vi "Parse XML.vi"(8 "error in (no error)":errorcluster, 10 "xml string":string) -> (0 "error out":errorcluster, 3 "xml out":T1)   [LabVIEW 2011]
uses:
  XML Structure - Cluster.ctl
  XML Tag Type - Enum.ctl
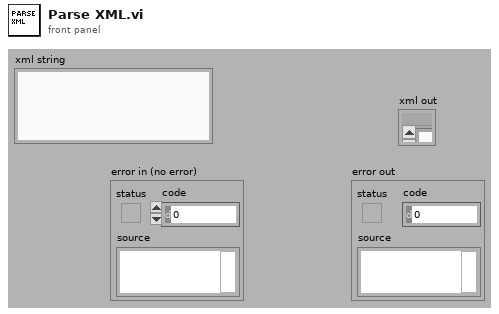
[diagram p1: front panel]
types:
  T1 = typedef "XML Structure - Cluster.ctl" = cluster{"tags":string[], "tag names":string[], "tag type":T2[], "offset":i32[], "close tag index":i32[], "xml":string, "Children":cluster{"children":i32[]}[], "parent index":i32[]}
  T2 = typedef "XML Tag Type - Enum.ctl" = enum16{"start tag", "empty tag", "end tag"}
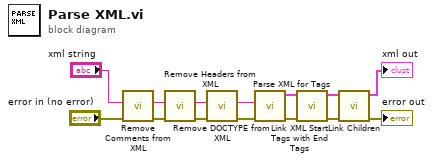
[diagram p0: block diagram]
diagram:
  n1 = call "Remove Comments from XML.vi"("error in (no error)"="error in (no error)", "XML (with comments)"="xml string") -> ("error out"=w5:errorcluster, "XML (without comments)"=w6:string)  [unwired: 8 in]
  n2 = call "Remove Headers from XML.vi"("error in (no error)"=w5, "XML (with headers)"=w6) -> ("error out"=w4:errorcluster, "XML (without headers)"=w2:string)  [unwired: 8 in]
  n3 = call "Remove DOCTYPE from XML.vi"("error in (no error)"=w4, "XML (with DOCTYPE)"=w2) -> ("error out"=w3:errorcluster, "XML (without DOCTYPE)"=w1:string)  [unwired: 7 in, 1 out]
  n4 = call "Parse XML for Tags.vi"("error in (no error)"=w3, "xml string"=w1) -> ("error out"=w12:errorcluster, "xml structure"=w11:T1)  [unwired: 8 in]
  n5 = call "Link XML Start Tags with End Tags.vi"("error in (no error)"=w12, "xml in"=w11) -> ("error out"=w8:errorcluster, "xml out"=w10:T1)  [unwired: 8 in]
  n6 = call "Link Children.vi"("error in (no error)"=w8, "xml structure"=w10) -> ("error out"=→"error out":errorcluster, "xml structure out"=→"xml out":T1)  [unwired: 8 in]
